vi "Find USB Device by Manufacturer.vi"(8 "error in (no error)":errorcluster, 11 "Match String":string) -> (0 "error out":errorcluster, 3 "reference out":refnum<visa-resource-name>)   [LabVIEW 2017]
panel:
  out "Array":string[](array[string])
  out "find list":string[](array[string])
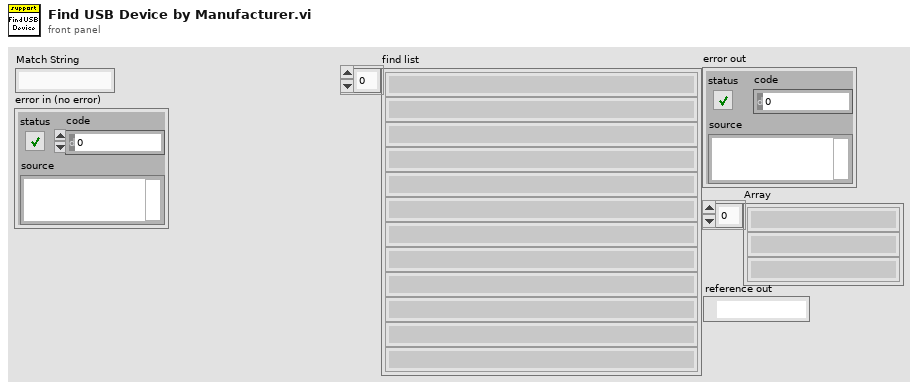
[diagram p1: front panel]
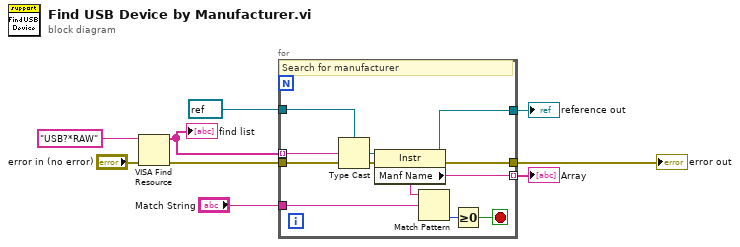
[diagram p0: block diagram]
diagram:
  n1 = VISA Find Resource(8:"error in (no error)", 11:"USB?*RAW" ("expression (\"?*\")")) -> (0:w2:errorcluster, 3:w8:string[])  [unwired: 1 in, 1 out]
  "find list" <- w8
  n2 = for {
    tunnel: w8 -> [w19] mode=indexing
    tunnel: [w17] -> w7 mode=indexing
    tunnel: "Match String" -> [w16]
    tunnel: refnum<visa-resource-name> refnum ("reference out") -> [w13]
    tunnel: [w12] -> w4
    tunnel: [w11] -> w3
    tunnel: w2 -> [w10]
    stop <- w15 stop-if-true
    # "Search for manufacturer"
    n3 = Type Cast(type=w13, x=w19) -> (*(type *) &x=w18:refnum<visa-resource-name>)
    n4 = property class="Instr"(reference=w18, error in=w10) -> (reference out=w11:refnum<visa-resource-name>, error out=w12:errorcluster, "Manf Name"=w17:string)
    n5 = Match Pattern(string=w17, regular expression=w16) -> (offset past match=w14:i32)  [unwired: 1 in, 3 out]
    n6 = Greater Or Equal To 0?(x=w14) -> (x >= 0?=w15:bool)
  }
  "error out" <- w4
  "Array" <- w7
  "reference out" <- w3
